vi "Setup Connector 0.vi"(11 "Bank Types":T1) -> (0 "Connector 0 Bank 3 out":refnum<class "Bank.lvclass">, 1 "Connector 0 Bank 2 out":refnum<class "Bank.lvclass">, 2 "Connector 0 Bank 1 out":refnum<class "Bank.lvclass">, 3 "Connector 0 Bank 0 out":refnum<class "Bank.lvclass">)   [LabVIEW 2019, in "LRUTS FPGA IP.lvlib"]
uses:
  Bank/Bank.lvclass
  Connector Bank Types.ctl
  Bank/Bank Type.ctl
  Bank List.ctl
  LRUTS FPGA IP.lvlib
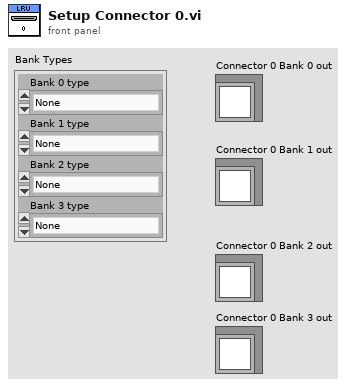
[diagram p1: front panel]
types:
  T1 = typedef "Connector Bank Types.ctl" = cluster{"Bank 0 type":T2, "Bank 1 type":T2, "Bank 2 type":T2, "Bank 3 type":T2}
  T2 = typedef "LRUTS FPGA IP.lvlib/Bank.lvclass/Bank Type.ctl" = enum16{"None", "Discrete Acquisition", "Discrete Generation", "PWM Acquisition", "PWM Generation"}
  T3 = typedef "LRUTS FPGA IP.lvlib/Bank List.ctl" = enum16{"Connector 0/Bank 0", "Connector 0/Bank 1", "Connector 0/Bank 2", "Connector 0/Bank 3", "Connector 1/Bank 0", "Connector 1/Bank 1", "Connector 1/Bank 2", "Connector 1/Bank 3", "Connector 2/Bank 0", "Connector 2/Bank 1", "Connector 2/Bank 2", "Connector 2/Bank 3", "Connector 3/Bank 0", "Connector 3/Bank 1", "Connector 3/Bank 2", "Connector 3/Bank 3"}
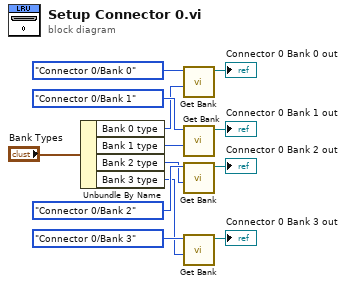
[diagram p0: block diagram]
diagram:
  n1 = Unbundle By Name("Bank Types") -> ("Bank 0 type"=w4:T2, "Bank 1 type"=w3:T2, "Bank 2 type"=w2:T2, "Bank 3 type"=w1:T2)
  n2 = call "Get Bank.vi"("Bank Type"=w4, 11:Bank_List."Connector 0/Bank 0") -> ("Bank out"=→"Connector 0 Bank 0 out":refnum<class "Bank.lvclass">)  [unwired: 9 in]
  n3 = call "Get Bank.vi"("Bank Type"=w3, 11:Bank_List."Connector 0/Bank 1") -> ("Bank out"=→"Connector 0 Bank 1 out":refnum<class "Bank.lvclass">)  [unwired: 9 in]
  n4 = call "Get Bank.vi"("Bank Type"=w2, 11:Bank_List."Connector 0/Bank 2") -> ("Bank out"=→"Connector 0 Bank 2 out":refnum<class "Bank.lvclass">)  [unwired: 9 in]
  n5 = call "Get Bank.vi"("Bank Type"=w1, 11:Bank_List."Connector 0/Bank 3") -> ("Bank out"=→"Connector 0 Bank 3 out":refnum<class "Bank.lvclass">)  [unwired: 9 in]
